vi "Stream Line (Polymorphic).vi"   [LabVIEW 2015, in "Zaber A Series.lvlib"]
doc: "Adds a line command to an open stream. The line will always start where the previous stream command leaves the device positioned. The endpoint can be specified relative to there, or in absolute coordinates. The endpoint is specified in microstep units - use the Convert Position to Device Units VI to convert from standard measurements.\n\nThis VI does not check in advance for error conditions such as streams not being supported or the stream not being open.\n\nThis VI requires that the Initialize VI has been called with the same serial port and that the specified stream is open."
uses:
  Zaber A Series.lvlib
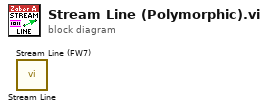
[diagram p0: block diagram]
diagram:
  n1 = call "Stream Line.vi"() -> ()  [unwired: 10 in, 2 out]
  n2 = call "Stream Line (FW7).vi"() -> ()  [unwired: 10 in, 2 out]
